vi "Scanner Read.vi"(8 "error in (no error)":errorcluster, 9 "Message Data":variant, 10 "Scanner notifier":refnum<notifier>, 11 "Hardware Resources in":T1={"Link"={"Connection"=enum."USB", "Host or IP address (TCP/IP)"="", "Port (Serial/USB)"="COM1"}, "VISA resource"="", "Writer Queue"=refnum, "Status"=FALSE}) -> (0 "error out":errorcluster, 1 "Message Data Out":variant, 3 "Hardware Resources out":T1={"Link"={"Connection"=enum."USB", "Host or IP address (TCP/IP)"="", "Port (Serial/USB)"="COM1"}, "VISA resource"="", "Writer Queue"=refnum, "Status"=FALSE})   [LabVIEW 2020, in "Hiden Scanner.lvlib"]
doc: "Perform the acquisition. Replace the contents of this diagram with calls to acquisition hardware."
uses:
  Hiden Scanner.lvlib
  support/Message Queue/Message Cluster.ctl
  support/Message Queue/Message Queue.lvlib
  Scanner Hardware Configuration.ctl
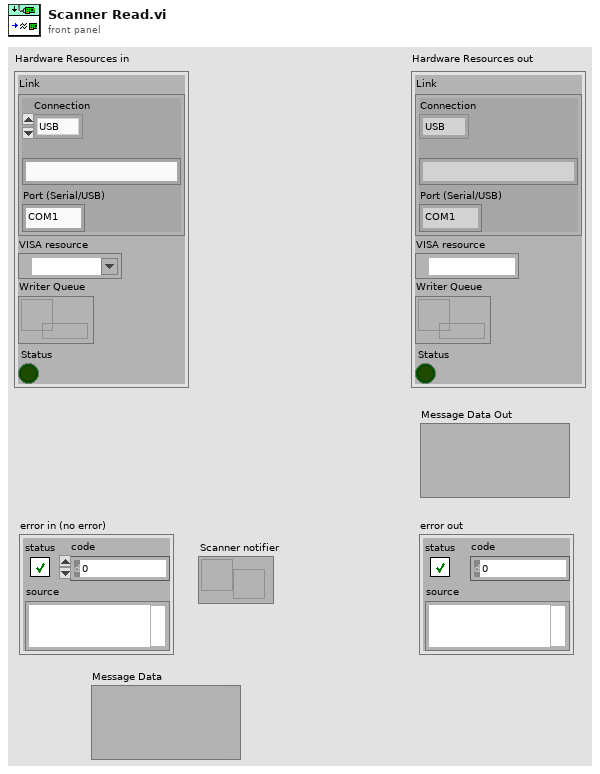
[diagram p1: front panel]
types:
  T1 = typedef "Hiden Scanner.lvlib/Scanner Hardware Configuration.ctl" = cluster{"Link":cluster{"Connection":enum16{"Serial", "TCP/IP", "USB"}, "Host or IP address (TCP/IP)":string, "Port (Serial/USB)":string}, "VISA resource":refnum<visa-resource-name>, "Writer Queue":refnum<queue>, "Status":bool}
  T2 = typedef "Message Queue.lvlib/Message Cluster.ctl" = cluster{"Message":string, "Message Data":variant}
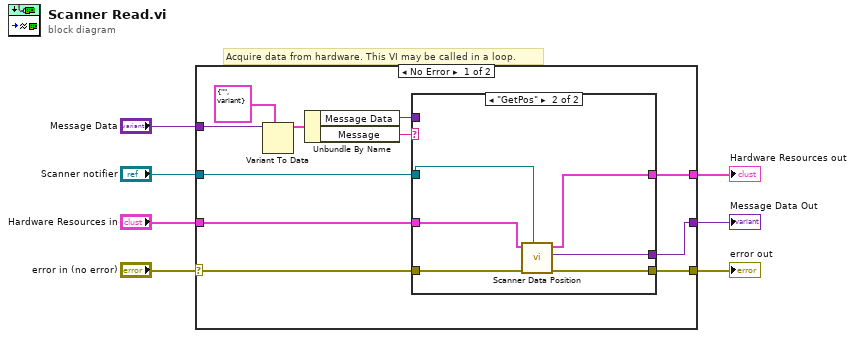
[diagram p0: block diagram]
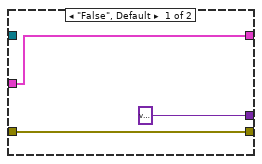
[diagram p2: hidden frame]
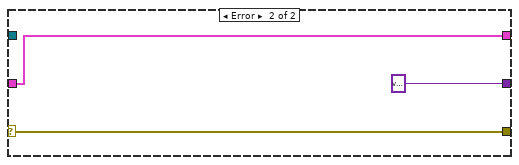
[diagram p3: hidden frame]
diagram:
  # "Acquire data from hardware. This VI may be called in a loop."
  n1 = case shown="No Error" "error in (no error)" {
    selector: "error in (no error)" -> [w18 w29]
    tunnel: [w15 w29] -> w6
    tunnel: "Hardware Resources in" -> [w17 w30]
    tunnel: [w16 w30] -> w4
    tunnel: [w14 variant ("Message Data Out")] -> w3
    tunnel: "Scanner notifier" -> [w11 _]
    tunnel: "Message Data" -> [w10 _]
    frame No Error {
      n2 = Variant To Data(type=T2 {"Message"="", "Message Data"=variant} ("element"), Variant=w10) -> (data=w12:T2)  [unwired: 1 in, 1 out]
      n3 = Unbundle By Name(w12) -> ("Message Data"=w8:variant, "Message"=w9:string)
      n4 = case shown="\"GetPos\"" w9 {
        tunnel: w18 -> [w20 w27]
        tunnel: w17 -> [w21 w26]
        tunnel: [w21 w25] -> w16
        tunnel: [w20 w24] -> w15
        tunnel: [variant ("Message Data Out") w23] -> w14
        tunnel: w11 -> [_ w22]
        tunnel: w8 -> [_ _]
        frame "False", Default {
        }
        frame "GetPos" {
          n5 = call "Scanner Data Position.vi"(7:w22, "error in (no error)"=w27, "Hardware Resources in"=w26) -> ("error out"=w24:errorcluster, "Message Data Out"=w23:variant, "Hardware Resources out"=w25:T1)  [unwired: 6 in]
        }
      }
    }
    frame Error {
    }
  }
  "Hardware Resources out" <- w4
  "error out" <- w6
  "Message Data Out" <- w3
